vi "Create Work Endpoints.vi"(4 "Special Terminals":T1={"Action"=-1, "Init"=-1, "Tag"=-1, "State in"=-1, "State out"=-1, "Error"=-1}, 8 "error in (no error)":errorcluster, 10 "Grouped Terminals":T3, 11 "Refs in":T2) -> (0 "error out":errorcluster, 3 "Refs":T2)   [LabVIEW 2020, in "FlexBlocks.lvlib"]
uses:
  FlexBlocks.lvlib
  Grouped Terminals.ctl
  Terminal Group.ctl
  Terminal Config.ctl
  Type Descriptor.ctl
  Terminal Direction.ctl
  Value Mode.ctl
  Special Terminal.ctl
  Terminal Mode.ctl
  Scripting Refs.ctl
  Special Terminal Indices.ctl
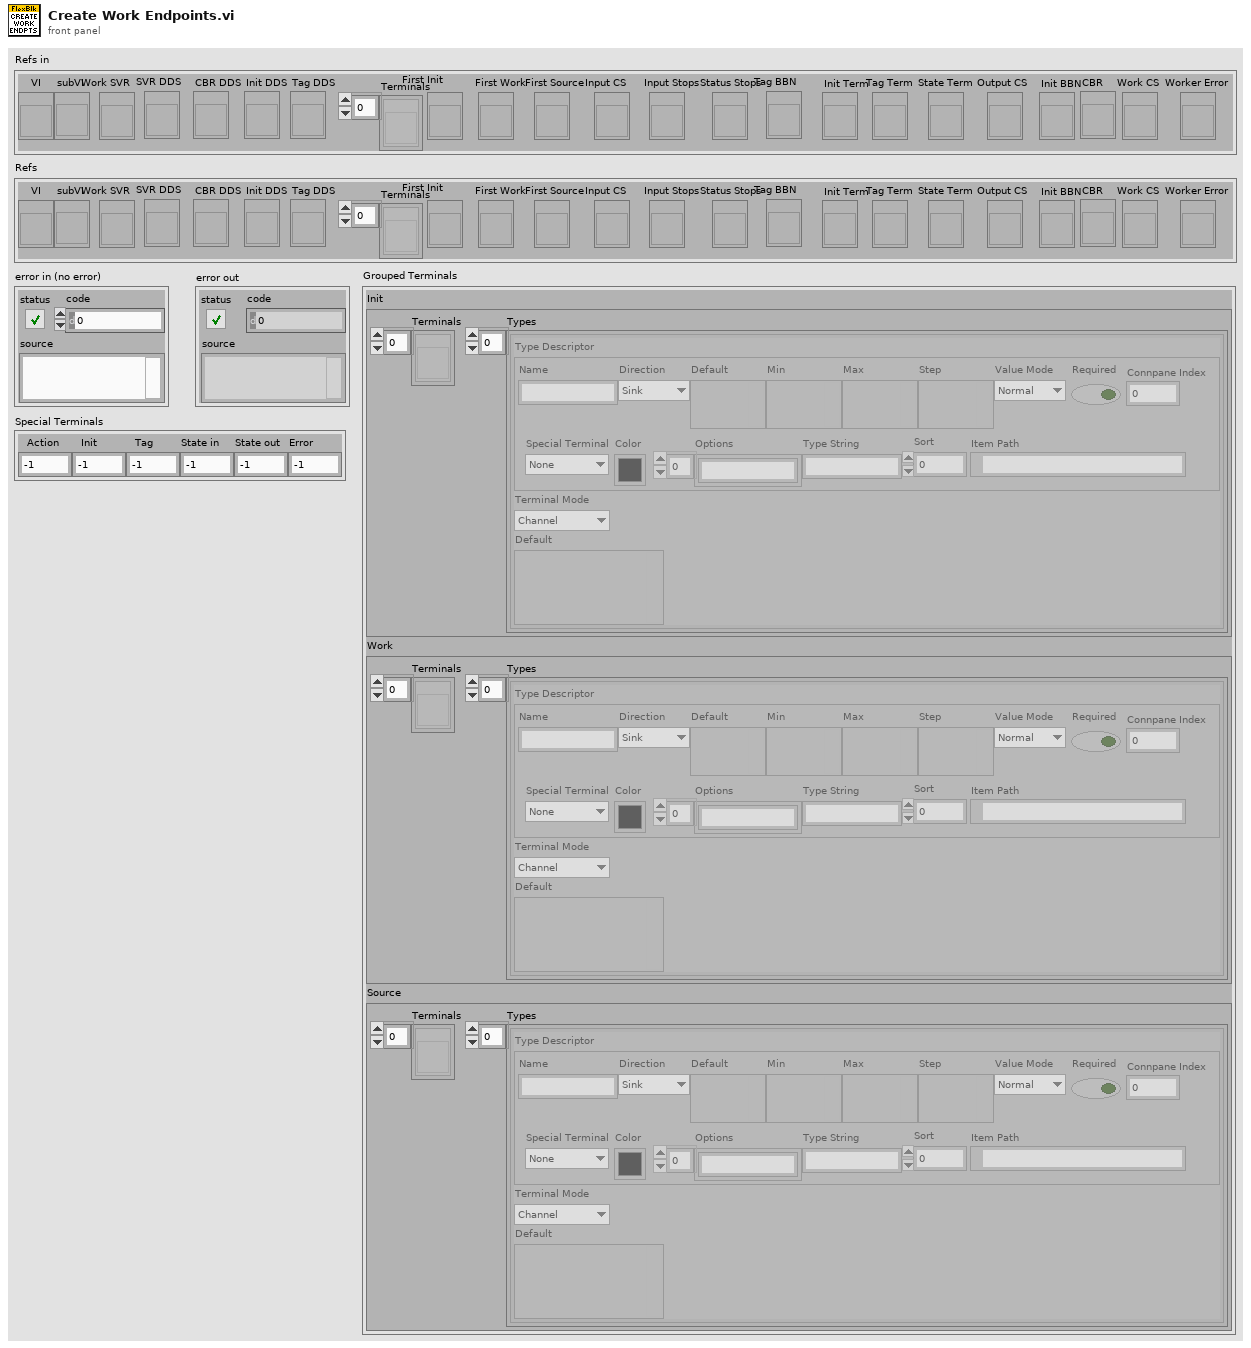
[diagram p1: front panel]
types:
  T1 = typedef "FlexBlocks.lvlib/Special Terminal Indices.ctl" = cluster{"Action":i32, "Init":i32, "Tag":i32, "State in":i32, "State out":i32, "Error":i32}
  T2 = typedef "FlexBlocks.lvlib/Scripting Refs.ctl" = cluster{"VI":refnum<vi>, "subVI":refnum<vi>, "Work SVR":refnum<vi>, "SVR DDS":refnum<vi>, "CBR DDS":refnum<vi>, "Init DDS":refnum<vi>, "Tag DDS":refnum<vi>, "Terminals":refnum<vi>[], "First Init":refnum<vi>, "First Work":refnum<vi>, "First Source":refnum<vi>, "Input CS":refnum<vi>, "Input Stops":refnum<vi>, "Status Stops":refnum<vi>, "Tag BBN":refnum<vi>, "Init Term":refnum<vi>, "Tag Term":refnum<vi>, "State Term":refnum<vi>, "Output CS":refnum<vi>, "Init BBN":refnum<vi>, "CBR":refnum<vi>, "Work CS":refnum<vi>, "Worker Error":refnum<vi>}
  T3 = typedef "FlexBlocks.lvlib/Grouped Terminals.ctl" = cluster{"Init":T4, "Work":T4, "Source":T4}
  T4 = typedef "FlexBlocks.lvlib/Terminal Group.ctl" = cluster{"Terminals":refnum<vi>[], "Types":T5[]}
  T5 = typedef "FlexBlocks.lvlib/Terminal Config.ctl" = cluster{"Type Descriptor":T6, "Terminal Mode":T10, "Default":variant}
  T6 = typedef "FlexBlocks.lvlib/Type Descriptor.ctl" = cluster{"Name":string, "Direction":T7, "Default":variant, "Min":variant, "Max":variant, "Step":variant, "Value Mode":T8, "Required":bool, "Connpane Index":i32, "Special Terminal":T9, "Color":u32, "Options":string[], "Type String":string, "Sort":i32, "Item Path":path}
  T7 = typedef "FlexBlocks.lvlib/Terminal Direction.ctl" = enum16{"Sink", "Source"}
  T8 = typedef "FlexBlocks.lvlib/Value Mode.ctl" = enum16{"Normal", "Range", "Select"}
  T9 = typedef "FlexBlocks.lvlib/Special Terminal.ctl" = enum16{"None", "Action", "Init", "Tag", "State in", "State out", "Error"}
  T10 = typedef "FlexBlocks.lvlib/Terminal Mode.ctl" = enum16{"Channel", "Config", "Value", "Control Ref"}
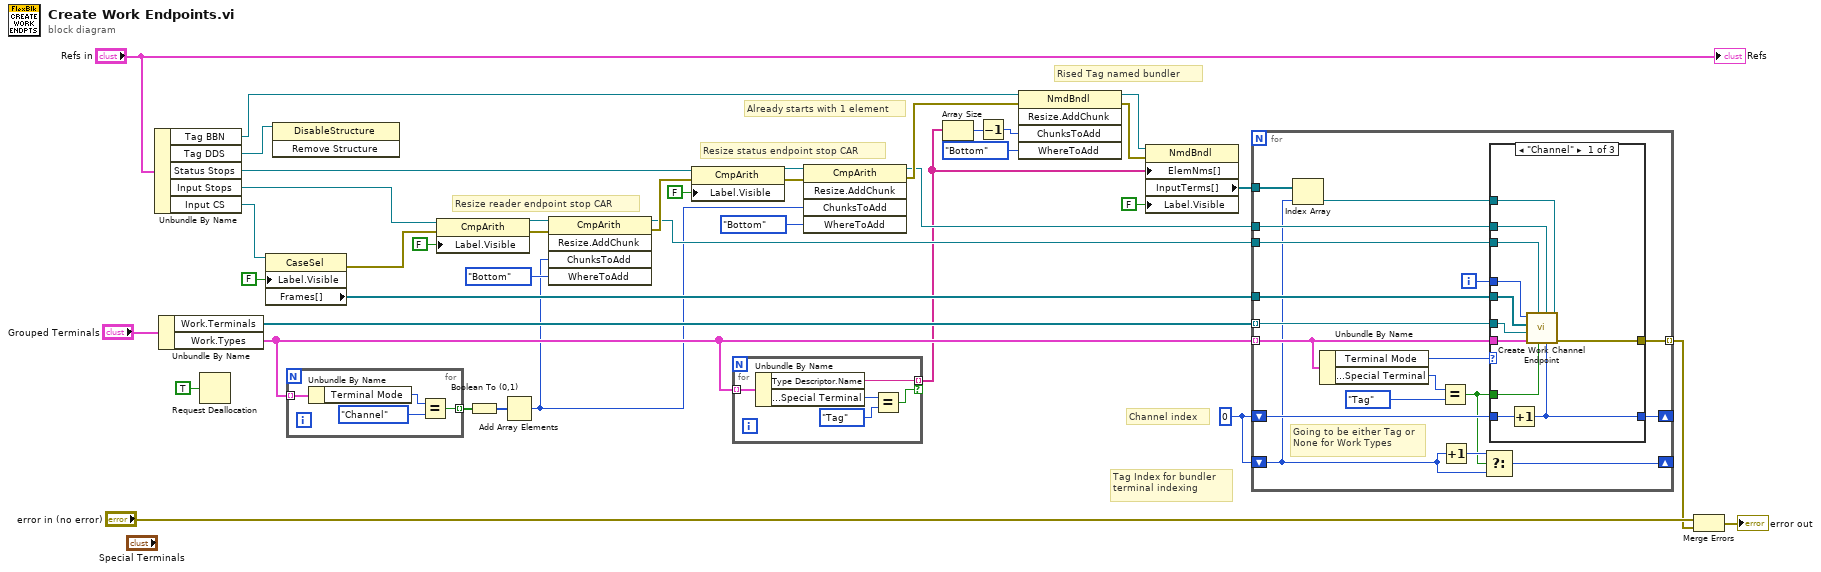
[diagram p0: block diagram]
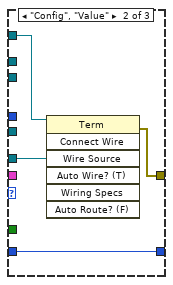
[diagram p2: hidden frame]
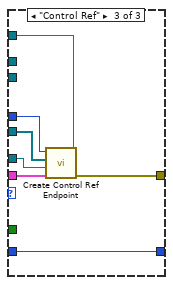
[diagram p3: hidden frame]
diagram:
  w1 = 0
  # "Tag Index for bundler terminal indexing"
  # "Channel index"
  # "Rised Tag named bundler"
  # "Resize status endpoint stop CAR"
  # "Resize reader endpoint stop CAR"
  # "Already starts with 1 element"
  n1 = Unbundle By Name("Refs in") -> ("Tag BBN"=w4:refnum<vi>, "Tag DDS"=w5:refnum<vi>, "Status Stops"=w6:refnum<vi>, "Input Stops"=w8:refnum<vi>, "Input CS"=w9:refnum<vi>)
  n2 = Unbundle By Name("Grouped Terminals") -> ("Work.Terminals"=w16:refnum<vi>[], "Work.Types"=w12:T5[])
  n3 = Request Deallocation(TRUE ("flag")) -> ()
  n4 = property class="CaseSel"(reference=w9, "Label.Visible"=FALSE) -> (error out=w7:errorcluster, "Frames[]"=w20:refnum<vi>[])  [unwired: 1 in, 1 out]
  n5 = invoke class="DisableStructure" method="Remove Structure"(reference=w5) -> ()  [unwired: 2 in, 3 out]
  n6 = for {
    tunnel: w12 -> [w44] mode=indexing
    tunnel: [w41] -> w32 mode=indexing
    n7 = Unbundle By Name(w44) -> ("Terminal Mode"=w43:T10)
    n8 = Equal?(x=w43, y=Terminal_Mode."Channel") -> (x = y?=w41:bool)
  }
  n9 = property class="CmpArith"(reference=w8, error in=w7, "Label.Visible"=FALSE) -> (reference out=w29:refnum<vi>, error out=w27:errorcluster)
  n10 = Boolean To (0,1)(Boolean=w32) -> (0, 1=w31:i16[])
  n11 = Add Array Elements(numeric array=w31) -> (sum=w2:i16)
  n12 = invoke class="CmpArith" method="Resize.AddChunk"(reference=w29, error in=w27, "ChunksToAdd"=w2, "WhereToAdd"=enum8{"Bottom", "Top"}."Bottom" ("Where To Add")) -> (reference out=w26:refnum<vi>, error out=w39:errorcluster)  [unwired: 1 in, 3 out]
  n13 = property class="CmpArith"(reference=w6, error in=w39, "Label.Visible"=FALSE) -> (reference out=w23:refnum<vi>, error out=w25:errorcluster)
  n14 = for {
    tunnel: w12 -> [w49] mode=indexing
    tunnel: [w46] -> w11 mode=indexing if=w45
    n15 = Unbundle By Name(w49) -> ("Type Descriptor.Name"=w46:string, "Type Descriptor.Special Terminal"=w48:T9)
    n16 = Equal?(x=w48, y=Special_Terminal."Tag") -> (x = y?=w45:bool)
  }
  n17 = invoke class="CmpArith" method="Resize.AddChunk"(reference=w23, error in=w25, "ChunksToAdd"=w2, "WhereToAdd"=enum8{"Bottom", "Top"}."Bottom" ("Where To Add")) -> (reference out=w21:refnum<vi>, error out=w40:errorcluster)  [unwired: 1 in, 3 out]
  n18 = Array Size(array=w11) -> (size(s)=w18:i32)
  n19 = Decrement(x=w18) -> (x-1=w17:i32)
  n20 = invoke class="NmdBndl" method="Resize.AddChunk"(reference=w4, error in=w40, "ChunksToAdd"=w17, "WhereToAdd"=enum8{"Bottom", "Top"}."Bottom" ("Where To Add")) -> (reference out=w15:refnum<vi>, error out=w14:errorcluster)  [unwired: 1 in, 3 out]
  n21 = property class="NmdBndl"(reference=w15, error in=w14, "ElemNms[]"=w11, "Label.Visible"=FALSE) -> ("InputTerms[]"=w10:refnum<vi>[])  [unwired: 2 out]
  n22 = for {
    tunnel: w16 -> [w67] mode=indexing
    tunnel: w12 -> [w62] mode=indexing
    tunnel: w20 -> [w63]
    tunnel: [w61] -> w33 mode=indexing
    tunnel: w26 -> [w59]
    tunnel: w21 -> [w58]
    shift-right: [w56] -> _
    shift-left: w1 -> [w57]
    tunnel: w10 -> [w55]
    shift-right: [w53] -> _
    shift-left: w1 -> [w51]
    i -> [w60]
    # "Going to be either Tag or None for Work Types"
    n23 = Index Array(array=w55, index=w51) -> (element=w52:refnum<vi>)
    n24 = Unbundle By Name(w62) -> ("Terminal Mode"=w64:T10, "Type Descriptor.Special Terminal"=w66:T9)
    n25 = Equal?(x=w66, y=Special_Terminal."Tag") -> (x = y?=w50:bool)
    n26 = Increment(x=w51) -> (x+1=w54:i32)
    n27 = Select(t=w54, s=w50, f=w51) -> (s? t:f=w53:i32)
    n28 = case shown="\"Channel\"" w64 {
      tunnel: w50 -> [w70 _ _]
      tunnel: w63 -> [w77 _ w85]
      tunnel: w62 -> [w71 _ w88]
      tunnel: w67 -> [w78 w81 w86]
      tunnel: [w68 w80 w87] -> w61
      tunnel: w60 -> [w76 _ w84]
      tunnel: w59 -> [w74 _ _]
      tunnel: w58 -> [w73 _ _]
      tunnel: w57 -> [w75 w82 w89]
      tunnel: [w69 w82 w89] -> w56
      tunnel: w52 -> [w72 w79 w83]
      frame "Channel" {
        n29 = Increment(x=w75) -> (x+1=w69:i32)
        n30 = call "Create Work Channel Endpoint.vi"("Bundler Terminal"=w72, "Channel Index"=w69, "Status CAR"=w73, "Lossy"=w70, "Input CAR"=w74, "Terminal Config"=w71, "Terminal"=w78, "Frames[]"=w77, "Index"=w76) -> ("error out"=w68:errorcluster)  [unwired: 2 in]
      }
      frame "Config", "Value" {
        n31 = invoke class="Term" method="Connect Wire"(reference=w79, "Wire Source"=w81) -> (error out=w80:errorcluster)  [unwired: 5 in, 6 out]
      }
      frame "Control Ref" {
        n32 = call "Create Control Ref Endpoint.vi"("Bundler Terminal"=w83, "Terminal Config"=w88, "Terminal"=w86, "Frames[]"=w85, "Index"=w84) -> ("error out"=w87:errorcluster)  [unwired: 6 in]
      }
    }
  }
  n33 = Merge Errors("error in (no error)", w33) -> (→"error out":errorcluster)
  "Refs" <- "Refs in"
